vi "Begin.vi"(8 "error in (no error)":errorcluster, 11 "Shifter in":refnum<class "Shifter.lvclass">) -> (0 "error out":errorcluster, 3 "Shifter out":refnum<class "Shifter.lvclass">)   [LabVIEW 2013, in "Shifter.lvclass"]
uses:
  Shifter.lvclass
  <vilib>/Rock Robotics/SystemInterfaces/Typedef/FPGA_TypedefSolenoidModule.ctl
  <vilib>/Rock Robotics/WPI/Solenoid/WPI_SolenoidChannel.ctl
  System/System.lvclass
  <vilib>/Rock Robotics/WPI/Solenoid/WPI_SolenoidOpenSingle.vi
panel:
  in  "Solenoid Channel":T1=enum."Solenoid 4"
  in  "Solenoid Module (Module 1)":T2
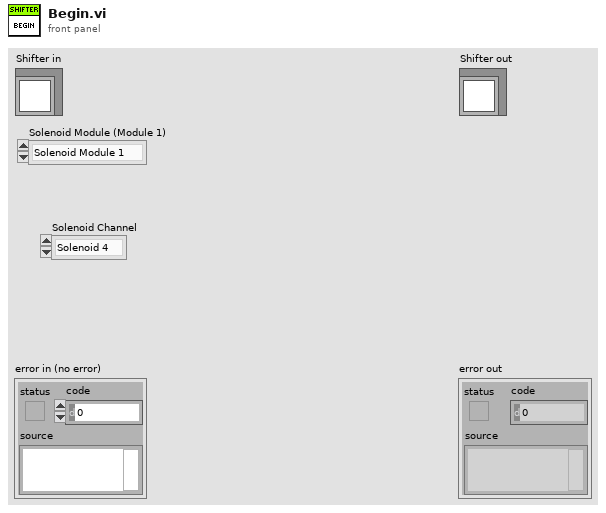
[diagram p1: front panel]
types:
  T1 = typedef "WPI_SolenoidChannel.ctl" = enum8{"Solenoid 1", "Solenoid 2", "Solenoid 3", "Solenoid 4", "Solenoid 5", "Solenoid 6", "Solenoid 7", "Solenoid 8", "Invalid"}
  T2 = typedef "FPGA_TypedefSolenoidModule.ctl" = enum16{"Solenoid Module 1", "Solenoid Module 2"}
  T3 = typedef "WPI_SolenoidDevRef.ctl" = cluster{"DevStatus":errorcluster, "Solenoid Module":T2, "Forward Solenoid Channel":T1, "Reverse Solenoid Channel":T1}
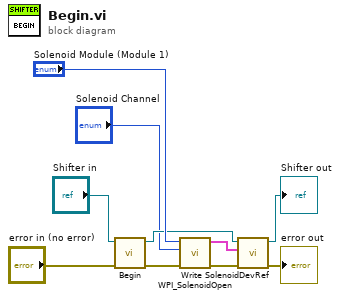
[diagram p0: block diagram]
diagram:
  n1 = call-parent "Begin.vi"("error in (no error)"="error in (no error)", "System in"="Shifter in") -> ("error out"=w2:errorcluster, "System out"=w6:refnum<class "Shifter.lvclass">)  [unwired: 8 in]
  n2 = call-poly <vilib>:"WPI_SolenoidOpen.vi"("error in (no error)"=w2, "Solenoid Channel"="Solenoid Channel", "Solenoid Module (Module 1)"="Solenoid Module (Module 1)") -> ("error out"=w3:errorcluster, "SolenoidDevRef"=w7:T3)  [unwired: 7 in]
  n3 = call-dynamic "Write SolenoidDevRef.vi"("error in (no error)"=w3, "SolenoidDevRef"=w7, "Shifter in"=w6) -> ("error out"=→"error out":errorcluster, "Shifter out"=→"Shifter out":refnum<class "Shifter.lvclass">)  [unwired: 7 in]
